vi "Phi_Theta 12 bit Merge.vi"(6 "Phi H/Theta H":u8, 7 "Theta L":u8, 8 "Phi L":u8) -> (0 "Theta":u16, 5 "Phi":u16)   [LabVIEW 2015]
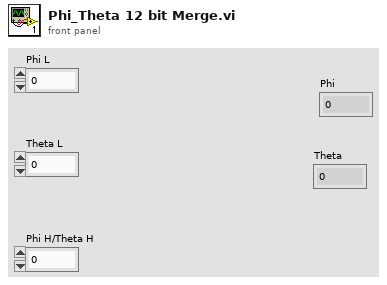
[diagram p1: front panel]
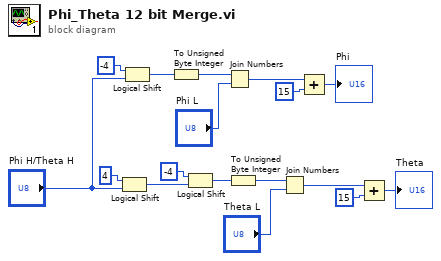
[diagram p0: block diagram]
diagram:
  n1 = Logical Shift(y=i16 4, x="Phi H/Theta H") -> (x << y=w8:u8)
  n2 = Logical Shift(y=i16 -4, x="Phi H/Theta H") -> (x << y=w10:u8)
  n3 = To Unsigned Byte Integer(number=w10) -> (unsigned 8bit integer=w15:u8)
  n4 = Logical Shift(y=i16 -4, x=w8) -> (x << y=w7:u8)
  n5 = Join Numbers(hi=w15, lo="Phi L") -> ((hi.lo)=w5:u16)
  n6 = To Unsigned Byte Integer(number=w7) -> (unsigned 8bit integer=w14:u8)
  n7 = Join Numbers(hi=w14, lo="Theta L") -> ((hi.lo)=w3:u16)
  n8 = Add(x=w5, y=u16 15) -> (x+y=→"Phi":u16)
  n9 = Add(x=w3, y=u16 15) -> (x+y=→"Theta":u16)
